vi "Do.vi"(7 "Mediated Asynchronous Actor":refnum<class "Mediated Asynchronous Actor.lvclass">, 8 "error in (no error)":errorcluster, 11 "Read Msg in":refnum<class "Read Msg.lvclass">) -> (0 "error out":errorcluster, 3 "Read Msg out":refnum<class "Read Msg.lvclass">, 5 "Mediated Asynchronous Actor out":refnum<class "Mediated Asynchronous Actor.lvclass">)   [LabVIEW 2016, in "Stream Mediator.lvlib" / "Read Msg.lvclass"]
doc: "--\nCopyright © 2017 Composed SystemsI All rights reserved.\n\nAuthor: Jon McBee <jon.mcbee@composed.io>\n\nThis library is provided \"AS IS\" ,WITHOUT WARRANTIES OR\nCONDITIONS OF ANY KIND, either express or implied.\n\nComposed Systems -- composed.io\n\nStream 0.0.1.1\nJon McBee - Composed Systems\nCopyright (c) 2017, Composed Systems"
uses:
  <userlib>/Composed Systems/Stream/Mediator/Classes/Websocket Client Handler Actor/Websocket Client Handler Msgs/Read Msg/Read Msg.lvclass
  <userlib>/Composed Systems/Stream/Mediator/Classes/Mediated Asynchronous Actor/Mediated Asynchronous Actor.lvclass
  <userlib>/Composed Systems/Stream/Mediator/Classes/Websocket Client Handler Actor/Websocket Client Handler/Websocket Client Handler.lvclass
  C:/Program Files (x86)/National Instruments/LabVIEW 2016/user.lib/Composed Systems/Stream/Mediator/Classes/Mediated Asynchronous Actor/Mediated Asynchronous Actor.lvclass
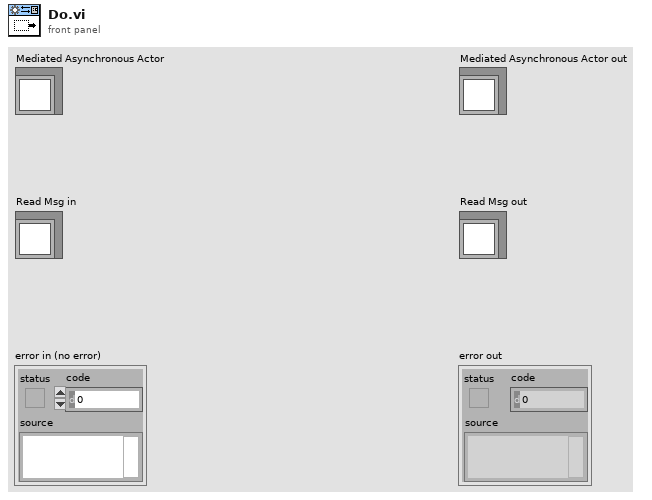
[diagram p1: front panel]
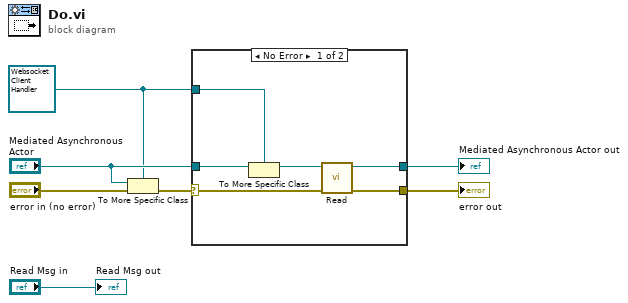
[diagram p0: block diagram]
diagram:
  w3 = refnum<class "Websocket Client Handler.lvclass"> refnum ("Websocket Client Handler.lvclass")
  n1 = To More Specific Class(target class=w3, reference="Mediated Asynchronous Actor", error in="error in (no error)") -> (error out=w6:errorcluster)  [unwired: 1 out]
  n2 = case shown="No Error" w6 {
    selector: w6 -> [w11 w14]
    tunnel: "Mediated Asynchronous Actor" -> [w13 w15]
    tunnel: w3 -> [w12 _]
    tunnel: [w9 w15] -> w2
    tunnel: [w8 w14] -> w1
    frame No Error {
      n3 = To More Specific Class(target class=w12, reference=w13) -> (specific class reference=w10:refnum<class "Websocket Client Handler.lvclass">)  [unwired: 1 in, 1 out]
      n4 = call <userlib>:"Read.vi"("error in (no error)"=w11, "Websocket Client Handler in"=w10) -> ("error out"=w8:errorcluster, "Websocket Client Handler out"=w9:refnum<class "Websocket Client Handler.lvclass">)  [unwired: 8 in]
    }
    frame Error {
    }
  }
  "error out" <- w1
  "Mediated Asynchronous Actor out" <- w2
  "Read Msg out" <- "Read Msg in"
